vi "JAVA_DriveConstants.vi"() -> ()   [LabVIEW 2016]
uses:
  TypeDef/CLUSTER_Drive_PIDF Constant.ctl
panel:
  out "PIDF Contants":T1
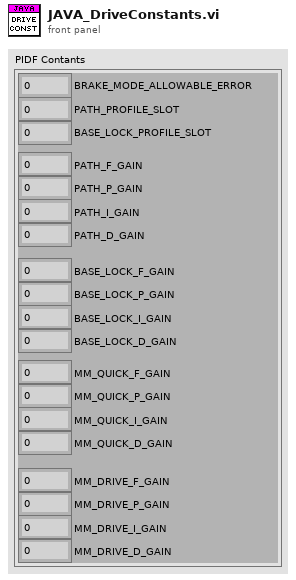
[diagram p1: front panel]
types:
  T1 = typedef "CLUSTER_Drive_PIDF Constant.ctl" = cluster{"BRAKE_MODE_ALLOWABLE_ERROR":i32, "PATH_PROFILE_SLOT":i32, "BASE_LOCK_PROFILE_SLOT":i32, "PATH_F_GAIN":dbl, "PATH_P_GAIN":dbl, "PATH_I_GAIN":dbl, "PATH_D_GAIN":dbl, "BASE_LOCK_F_GAIN":dbl, "BASE_LOCK_P_GAIN":dbl, "BASE_LOCK_I_GAIN":dbl, "BASE_LOCK_D_GAIN":dbl, "MM_QUICK_F_GAIN":dbl, "MM_QUICK_P_GAIN":dbl, "MM_QUICK_I_GAIN":dbl, "MM_QUICK_D_GAIN":dbl, "MM_DRIVE_F_GAIN":dbl, "MM_DRIVE_P_GAIN":dbl, "MM_DRIVE_I_GAIN":dbl, "MM_DRIVE_D_GAIN":dbl}
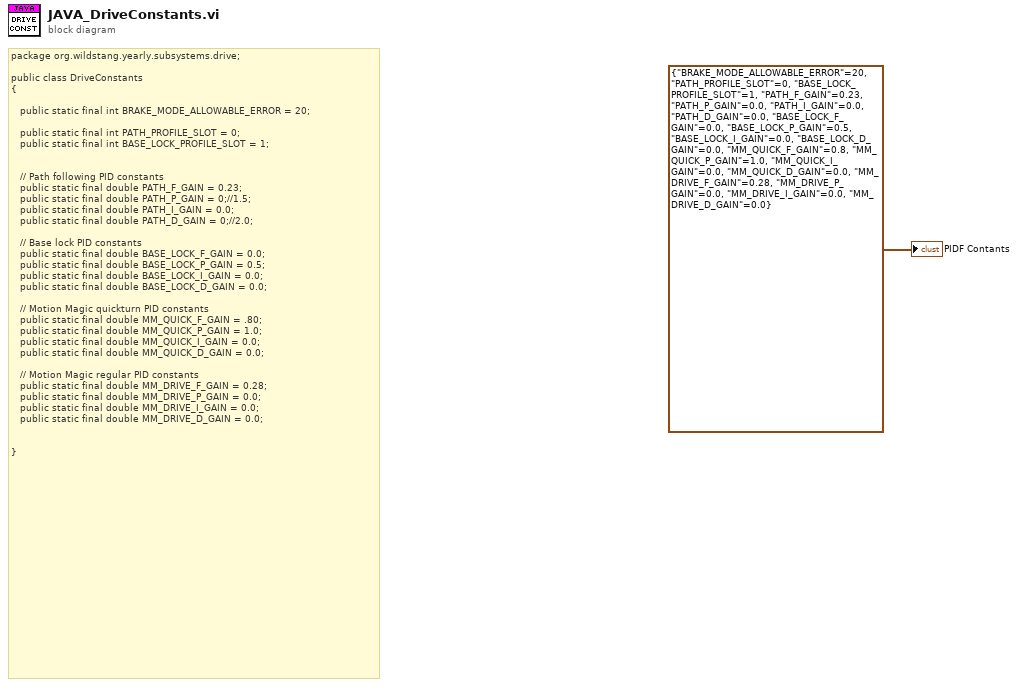
[diagram p0: block diagram]
diagram:
  # "package org.wildstang.yearly.subsystems.drive;\n\npublic class DriveConstants\n{\n\n   public static final int BRAKE_MODE_ALLOWABLE_ERROR = 20;\n   \n   public static final int PATH_PROFILE_SLOT = 0;\n   public static final int BASE_LOCK_PROFILE_SLOT = 1;\n   \n   \n   // Path following PID constants\n   public static final double PATH_F_GAIN = 0.23;\n   public static final double PATH_P_GAIN = 0;//1.5;\n   public static final double PATH_I_GAIN = 0.0;\n   public static final double PATH_D_GAIN = 0;//2.0;\n   \n   // Base lock PID constants\n   public static final double BASE_LOCK_F_GAIN = 0.0;\n   public static final double BASE_LOCK_P_GAIN = 0.5;\n   public static final double BASE_LOCK_I_GAIN = 0.0;\n   public static final double BASE_LOCK_D_GAIN = 0.0;\n\n   // Motion Magic quickturn PID constants\n   public static final double MM_QUICK_F_GAIN = .80;\n   public static final double MM_QUICK_P_GAIN = 1.0;\n   public static final double MM_QUICK_I_GAIN = 0.0;\n   public static final double MM_QUICK_D_GAIN = 0.0;\n\n   // Motion Magic regular PID constants\n   public static final double MM_DRIVE_F_GAIN = 0.28;\n   public static final double MM_DRIVE_P_GAIN = 0.0;\n   public static final double MM_DRIVE_I_GAIN = 0.0;\n   public static final double MM_DRIVE_D_GAIN = 0.0;\n\n   \n}"
  "PIDF Contants" <- T1 {"BRAKE_MODE_ALLOWABLE_ERROR"=20, "PATH_PROFILE_SLOT"=0, "BASE_LOCK_PROFILE_SLOT"=1, "PATH_F_GAIN"=0.23, "PATH_P_GAIN"=0.0, "PATH_I_GAIN"=0.0, "PATH_D_GAIN"=0.0, "BASE_LOCK_F_GAIN"=0.0, "BASE_LOCK_P_GAIN"=0.5, "BASE_LOCK_I_GAIN"=0.0, "BASE_LOCK_D_GAIN"=0.0, "MM_QUICK_F_GAIN"=0.8, "MM_QUICK_P_GAIN"=1.0, "MM_QUICK_I_GAIN"=0.0, "MM_QUICK_D_GAIN"=0.0, "MM_DRIVE_F_GAIN"=0.28, "MM_DRIVE_P_GAIN"=0.0, "MM_DRIVE_I_GAIN"=0.0, "MM_DRIVE_D_GAIN"=0.0} ("PIDF Contants")
